vi "Check Path.vi"(8 "error in":errorcluster, 11 "Path":path) -> (0 "error out":errorcluster)   [LabVIEW 2018, in "TortoiseGit Show Log.lvlib"]
doc: "Merge in an error if the VI path is invalid e.g. the VI has not been saved."
uses:
  TortoiseGit Show Log.lvlib
  <vilib>/Utility/error.llb/Error Cluster From Error Code.vi
  <vilib>/ErrorRing/Error Ring.xnode
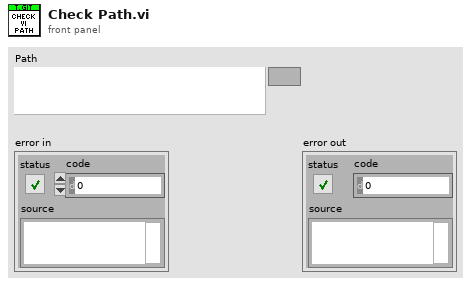
[diagram p1: front panel]
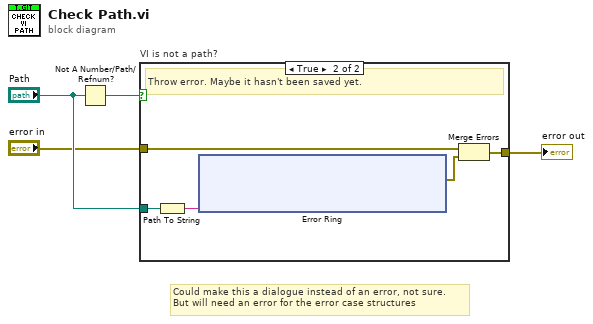
[diagram p0: block diagram]
diagram:
  # "Could make this a dialogue instead of an error, not sure.\nBut will need an error for the error case structures"
  n1 = Not A Number/Path/Refnum?(number/path/refnum="Path") -> (NaN/Path/Refnum?=w1:bool)
  n2 = case "VI is not a path?" shown="True" w1 {
    tunnel: [w5 w9] -> w3
    tunnel: "Path" -> [_ w7]
    tunnel: "error in" -> [w5 w6]
    frame False {
      # "VI is a path: no need to error"
    }
    frame True {
      # "Throw error. Maybe it hasn't been saved yet."
      n3 = Path To String(path=w7) -> (string=w8:string)
      n4 = xnode "Error Ring"("parameter 0"=w8) -> ("error out"=w10:errorcluster)
      n5 = Merge Errors(w6, w10) -> (w9:errorcluster)
    }
  }
  "error out" <- w3
